vi "PH_Beamline.color LL BL.vi"(0 "i ref in":refnum<vi>, 2 "Color State Exp LB Input":i32, 5 "error in (no error)":errorcluster) -> (14 "i ref out":refnum<vi>, 19 "error out":errorcluster)   [LabVIEW 2014, in "PH_Beamline.lvlib"]
doc: "This Vi colors the Laserlabor beamline elements."
uses:
  PH_Beamline.lvlib
  PH_Basics/PH_StatusHandler/PH_StatusHandler.Status.ctl
  PH_Basics/PH_Common/PH_Common.lvlib
  PH_BL-Master/PH_BL-Master.lvlib
  PH_Basics/PH_StatusHandler/PH_StatusHandler.lvlib
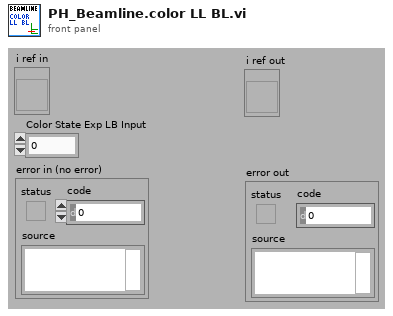
[diagram p1: front panel]
types:
  T1 = typedef "PH_StatusHandler.lvlib/PH_StatusHandler.Status.ctl" = i16
  T2 = typedef "PH_Beamline.lvlib/PH_Beamline.i attribute.ctl" = cluster{"GUI Refs":cluster{"PA ok":refnum<vi>, "MA ok":refnum<vi>, "fs FE ok":refnum<vi>, "ns FE ok":refnum<vi>, "PA ED ok":refnum<vi>, "MAS ok":refnum<vi>, "Booster ok":refnum<vi>, "Mirrortower ok":refnum<vi>, "In.-Box ok":refnum<vi>, "Compressor ok":refnum<vi>, "Experiment LB ok":refnum<vi>, "Experiment LL ok":refnum<vi>, "PHELIX_Beckhoff_Watchdog":refnum<vi>, "Shutters closed":refnum<vi>, "uOPA ok":refnum<vi>, "Vacuum no shotcond Comp LB":refnum<vi>}, "Refs BL MA":refnum<vi>[], "Refs BL MA-IB":refnum<vi>[], "Refs BL fs":refnum<vi>[], "Refs BL PA ED":refnum<vi>[], "Refs BL MAS":refnum<vi>[], "Refs BL Boo":refnum<vi>[], "Refs BL ns":refnum<vi>[], "Refs BL Mirrortower":refnum<vi>[], "Refs BL Compressor":refnum<vi>[], "Refs BL Exp LB":refnum<vi>[], "Radiation Safety":cluster{"Exp Laserbay":cluster{"Ref Op Mode":refnum<vi>, "Ref Laserbay evacuated":refnum<vi>, "Tagname LB evacuated":string, "Shot Mode":T3, "Laserbay evacuated?":i32, "Tagname HV room locked":string, "HV room locked?":i32, "Ref HV room locked":refnum<vi>, "Tagname bridged?":string, "Ref Bridge":refnum<vi>, "I<1E18W/cm²":bool}, "Exp Laserlab":cluster{"Ref Op Mode":refnum<vi>, "Ref Laserlab evacuated":refnum<vi>, "Tagname LL evacuated":string, "Shot Mode":T3, "Laserlab evacuated?":i32, "Tagname bridged?":string, "Ref Bridge":refnum<vi>, "I<1E18W/cm²":bool}}, "Refs BL LL":refnum<vi>[], "PP Igni Heating GUI Refs":refnum<vi>[], "PP Igni Heating Tagnames ":string[], "Refs BL PA":cluster{"undelayed Line before Shutter":refnum<vi>[], "undelayed Line after Shutter":refnum<vi>[], "before Bypass":refnum<vi>[], "delayed Line before Shutter":refnum<vi>[], "delayed Line after Shutter":refnum<vi>[], "before Shutter Input":refnum<vi>[], "after Shutter Input":refnum<vi>[], "Bypass":refnum<vi>[], "before Shutter Exit":refnum<vi>[], "after Shutter Exit":refnum<vi>[], "to MA":refnum<vi>[], "to Lab":refnum<vi>[]}, "BL":cluster{"YLF_BL_Status":i32, "fs_BL_Status":i32, "fs_YLF_BL_Status":i32, "ns_BL_Status":i32, "PA_Input_BL_Status":i32, "PA_UnDelay_BL_Status":i32, "PA_Delay_BL_Status":i32, "PA_BL_Status":i32, "PA_Bypass_BL_Status":i32, "PA_Exit_BL_Status":i32, "PA_LL_BL_Status":i32, "LL_BL_Status":i32, "PA_MA_BL_Status":i32, "MA_Exit_BL_Status":i32, "MA_Z6_BL_Status":i32, "Z6_BL_Status":i32, "MA_LB_BL_Status":i32, "LB_TB2_BL_Status":i32, "PA_before_Bypass_BL_Status":i32, "LB_TB3_BL_Status":i32}, "State Subsystems":cluster{"PA":bool, "MA":bool, "ns FE":bool, "fs FE":bool, "PA ED":bool, "In.-Box":bool, "MAS":bool, "Booster":bool, "Mirrortower":bool, "Compressor":bool, "Experiment LB":bool, "Experiment LL":bool, "uOPA":bool}, "Status Subscriber Information":T4, "Refs BL uOPA":refnum<vi>[], "PA_Input_2_Beam_6PWpGUI not linked?":bool, "PA_Input_Delay_6PGUI not linked?":bool, "Settings":T7}
  T3 = typedef "PH_Beamline.lvlib/PH_Beamline.Operation Mode.ctl" = i32
  T4 = typedef "PH_Beamline.lvlib/PH_Beamline.Status Subscriber Information.ctl" = cluster{"fs Swich YLF":T5, "fs Exit Shutter":T5, "ns Exit Shutter":T5, "PA Input Shutter":T5, "PA PC WP":T5, "PA PC WP 2":T5, "PA Bypass In":T5, "PA Bypass Out":T5, "PA CH 1":T5, "PA delayed":T5, "PA non delayed":T5, "PA Exit Shutter":T5, "PA Switch Lab":T5, "PA Bridge CH Input MA":T5, "MA Diffusor IB":T5, "MA IB Ready":T5, "MA CH 1":T5, "MA CH 2":T5, "MA CH 3":T5, "MA CH 4":T5, "MA Shutter Align Cam":T5, "MA Position MM5":T5, "Calorimeter Switch":T5, "BL Z6 CH 9":T5, "BL Z6 Beamdump":T5, "BL Z6 Shutter":T5, "COS Sensitivity Switch":T5, "Exp LB Shutter":T5, "Exp LB TB 2":T5, "Exp LB TB 3":T5, "PA LL Input CH":T5, "PA LL Output CH":T5, "LL Comp Input Shutter":T5, "LL Comp Output Shutter":T5, "LL Comp FF Shutter":T5, "Exp LL Shutter":T5, "MA IM In IB":T5, "MA IM Out IB":T5, "MA DB In IB":T5, "MA DB Out IB":T5, "Exp LB Shutter Interlock":T5, "Exp LL Shutter Interlock":T5, "MM1 Force Sensor":T5}
  T5 = typedef "PH_BL-Master.lvlib/PH_BL-Master.Status Subscriber Information.ctl" = cluster{"Index of element":i32, "Attributeset":T6}
  T6 = typedef "PH_BL-Master.lvlib/PH_BL-Master.Attribute Set.ctl" = enum16{"Boolean Status Service Subscriber", "Picture Status Service Subscriber"}
  T7 = typedef "PH_Beamline_Chief.lvlib/PH_Beamline_Chief.Settings.ctl" = cluster{"PA Doublepass Mode":bool, "Compressor Vaccuum LB not relevant":bool, "Windowshutter TB2 not relevant":bool, "Windowshutter TB3 not relevant":bool}
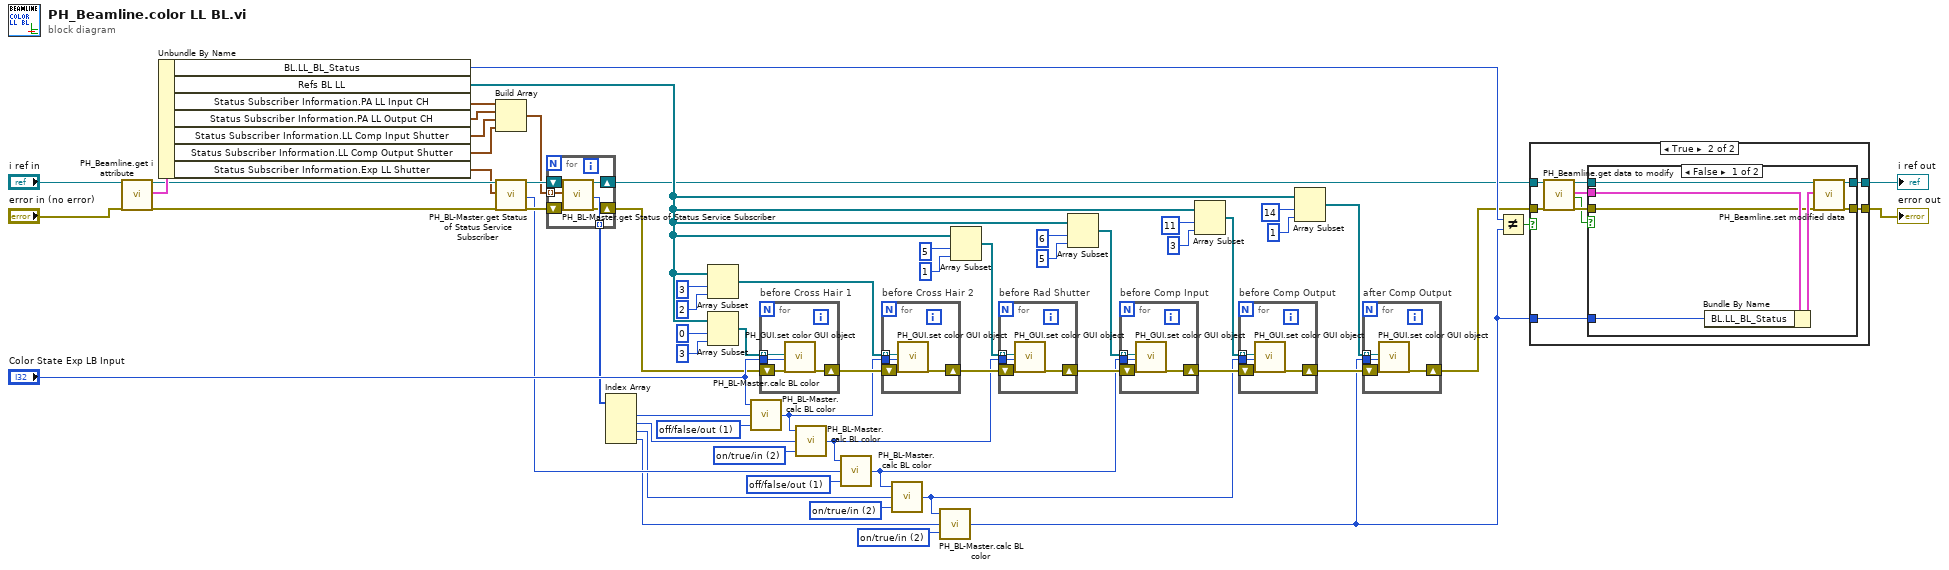
[diagram p0: block diagram]
diagram:
  w15 = T1 2 items=["no info", "off/false/out", "on/true/in", "Failure", "Alarm", "Status 1", "Status 2", "Status 3"] ("State for \"2\" (on) of ABLE (off/false/out)")
  w28 = T1 2 items=["no info", "off/false/out", "on/true/in", "Failure", "Alarm", "Status 1", "Status 2", "Status 3"] ("State for \"2\" (on) of ABLE (off/false/out)")
  w34 = T1 1 items=["no info", "off/false/out", "on/true/in", "Failure", "Alarm", "Status 1", "Status 2", "Status 3"] ("State for \"2\" (on) of ABLE (off/false/out)")
  w48 = T1 1 items=["no info", "off/false/out", "on/true/in", "Failure", "Alarm", "Status 1", "Status 2", "Status 3"] ("State for \"2\" (on) of ABLE (off/false/out)")
  w49 = T1 2 items=["no info", "off/false/out", "on/true/in", "Failure", "Alarm", "Status 1", "Status 2", "Status 3"] ("State for \"2\" (on) of ABLE (off/false/out)")
  n1 = call "PH_Beamline.get i attribute.vi"("i ref in"="i ref in", "error in (no error)"="error in (no error)") -> ("i ref out"=w10:refnum<vi>, "i attribute"=w61:T2, "error out"=w9:errorcluster)  [unwired: 15 in]
  n2 = Unbundle By Name(w61) -> ("BL.LL_BL_Status"=w42:i32, "Refs BL LL"=w18:refnum<vi>[], "Status Subscriber Information.PA LL Input CH"=w5:T5, "Status Subscriber Information.PA LL Output CH"=w4:T5, "Status Subscriber Information.LL Comp Input Shutter"=w3:T5, "Status Subscriber Information.LL Comp Output Shutter"=w2:T5, "Status Subscriber Information.Exp LL Shutter"=w6:T5)
  n3 = Build Array(w5, w4, w3, w2) -> (w1:T5[])
  n4 = call "PH_BL-Master.get Status of Status Service Subscriber.vi"("i ref in"=w10, "Wanted Status Subscriber Information"=w6, "error in (no error)"=w9) -> ("i ref out"=w47:refnum<vi>, "Status"=w33:T1, "error out"=w46:errorcluster)  [unwired: 11 in, 3 out]
  n5 = for {
    tunnel: [w67] -> w31 mode=indexing
    shift-right: [w66] -> w8
    shift-left: w47 -> [w64]
    shift-right: [w65] -> w7
    shift-left: w46 -> [w63]
    tunnel: w1 -> [w62] mode=indexing
    n6 = call "PH_BL-Master.get Status of Status Service Subscriber.vi"("i ref in"=w64, "Wanted Status Subscriber Information"=w62, "error in (no error)"=w63) -> ("i ref out"=w66:refnum<vi>, "Status"=w67:T1, "error out"=w65:errorcluster)  [unwired: 11 in, 3 out]
  }
  n7 = Index Array(array=w31) -> (element #1=w32:T1, element #2=w30:T1, element #3=w27:T1, element #4=w16:T1)  [unwired: 4 in]
  n8 = Array Subset(array=w18, index=3 ("length"), length=2) -> (w52:refnum<vi>[])
  n9 = Array Subset(array=w18, index=0, length=3) -> (w60:refnum<vi>[])
  n10 = call "PH_BL-Master.calc BL color.vi"("State for \"2\" (on) of ABLE (off/false/out)"=w48, "State ABLE"=w32, "State before ABLE"="Color State Exp LB Input") -> ("State after ABLE"=w50:i32)
  n11 = for "before Cross Hair 1" {
    tunnel: w60 -> [w71] mode=indexing
    shift-right: [w69] -> w55
    shift-left: w7 -> [w70]
    tunnel: "Color State Exp LB Input" -> [w68]
    n12 = call "PH_GUI.set color GUI object.vi"("GUI object Ref"=w71, "State"=w68, "error in (no error)"=w70) -> ("error out"=w69:errorcluster)  [unwired: 16 in]
  }
  n13 = call "PH_BL-Master.calc BL color.vi"("State for \"2\" (on) of ABLE (off/false/out)"=w49, "State ABLE"=w30, "State before ABLE"=w50) -> ("State after ABLE"=w35:i32)
  n14 = call "PH_BL-Master.calc BL color.vi"("State for \"2\" (on) of ABLE (off/false/out)"=w34, "State ABLE"=w33, "State before ABLE"=w35) -> ("State after ABLE"=w29:i32)
  n15 = for "before Cross Hair 2" {
    tunnel: w52 -> [w75] mode=indexing
    shift-right: [w73] -> w41
    shift-left: w55 -> [w74]
    tunnel: w50 -> [w72]
    n16 = call "PH_GUI.set color GUI object.vi"("GUI object Ref"=w75, "State"=w72, "error in (no error)"=w74) -> ("error out"=w73:errorcluster)  [unwired: 16 in]
  }
  n17 = call "PH_BL-Master.calc BL color.vi"("State for \"2\" (on) of ABLE (off/false/out)"=w28, "State ABLE"=w27, "State before ABLE"=w29) -> ("State after ABLE"=w14:i32)
  n18 = call "PH_BL-Master.calc BL color.vi"("State for \"2\" (on) of ABLE (off/false/out)"=w15, "State ABLE"=w16, "State before ABLE"=w14) -> ("State after ABLE"=w13:i32)
  n19 = Array Subset(array=w18, index=5 ("length"), length=1) -> (w39:refnum<vi>[])
  n20 = for "before Rad Shutter" {
    tunnel: w39 -> [w79] mode=indexing
    shift-right: [w77] -> w40
    shift-left: w41 -> [w78]
    tunnel: w35 -> [w76]
    n21 = call "PH_GUI.set color GUI object.vi"("GUI object Ref"=w79, "State"=w76, "error in (no error)"=w78) -> ("error out"=w77:errorcluster)  [unwired: 16 in]
  }
  n22 = Array Subset(array=w18, index=6 ("length"), length=5) -> (w36:refnum<vi>[])
  n23 = for "before Comp Input" {
    tunnel: w36 -> [w83] mode=indexing
    shift-right: [w81] -> w23
    shift-left: w40 -> [w82]
    tunnel: w29 -> [w80]
    n24 = call "PH_GUI.set color GUI object.vi"("GUI object Ref"=w83, "State"=w80, "error in (no error)"=w82) -> ("error out"=w81:errorcluster)  [unwired: 16 in]
  }
  n25 = Array Subset(array=w18, index=11 ("length"), length=3) -> (w24:refnum<vi>[])
  n26 = for "before Comp Output" {
    tunnel: w24 -> [w87] mode=indexing
    shift-right: [w85] -> w22
    shift-left: w23 -> [w86]
    tunnel: w14 -> [w84]
    n27 = call "PH_GUI.set color GUI object.vi"("GUI object Ref"=w87, "State"=w84, "error in (no error)"=w86) -> ("error out"=w85:errorcluster)  [unwired: 16 in]
  }
  n28 = Array Subset(array=w18, index=14 ("length"), length=1) -> (w17:refnum<vi>[])
  n29 = for "after Comp Output" {
    tunnel: w17 -> [w91] mode=indexing
    shift-right: [w89] -> w21
    shift-left: w22 -> [w90]
    tunnel: w13 -> [w88]
    n30 = call "PH_GUI.set color GUI object.vi"("GUI object Ref"=w91, "State"=w88, "error in (no error)"=w90) -> ("error out"=w89:errorcluster)  [unwired: 16 in]
  }
  n31 = Not Equal?(x=w42, y=w13) -> (x != y?=w45:bool)
  n32 = case shown="True" w45 {
    tunnel: w8 -> [w93 w98]
    tunnel: [w93 w97] -> w44
    tunnel: w21 -> [w92 w96]
    tunnel: [w92 w95] -> w43
    tunnel: w13 -> [_ w94]
    frame False {
    }
    frame True {
      n33 = call "PH_Beamline.get data to modify.vi"("i ref in"=w98, "error in (no error)"=w96) -> ("i ref out"=w101:refnum<vi>, "i attribute"=w99:T2, "timed out"=w100:bool, "error out"=w102:errorcluster)  [unwired: 14 in]
      n34 = case shown="False" w100 {
        tunnel: w102 -> [w103 w110]
        tunnel: w101 -> [w109 w111]
        tunnel: [w108 w110] -> w95
        tunnel: [w107 w111] -> w97
        tunnel: w99 -> [w104 _]
        tunnel: w94 -> [w105 _]
        frame False {
          n35 = Bundle By Name(cluster=w104, "BL.LL_BL_Status"=w105) -> (w106:T2)
          n36 = call "PH_Beamline.set modified data.vi"("i ref in"=w109, "i attribute"=w106, "error in (no error)"=w103) -> ("i ref out"=w107:refnum<vi>, "error out"=w108:errorcluster)  [unwired: 15 in]
        }
        frame True {
        }
      }
    }
  }
  "error out" <- w43
  "i ref out" <- w44
